vi "SHG_scattering_control.vi"() -> ()   [LabVIEW 2017]
uses:
  <instrlib>/Keithley 2200 Series/Keithley 2200 Series.lvlib
panel:
  in  "batch_bck location":path
  in  "batch_shg location":path
  in  "Take_bck_scan.exe location":path
  in  "Exposure Time (s)":dbl format="%#_13g"
  in  "Ouput Polarization (P_out OR S_out)":string
  in  "SHG_scat_scan.exe location":path
  in  "Power Supply":refnum<visa-resource-name>
  in  "Angle Resolution\n(Degrees per step)":i32
  in  "Min Angle":i32
  in  "Max Angle":i32
  in  "Number of Accum.":i32
  in  "S_in":bool=TRUE
  in  "P_in":bool=TRUE
  in  "System":string
  # "These file paths will be set to default positions"
  # "Data File parameters\n(Files save as: \nSystem_outputPol_inputPol_##_degrees_date)"
  # "Scan Inputs"
  # "The acceptable range is from\n-90 to 110 degrees"
  # "Polarizations to use (all nonrepetitive\n combinations will be scanned)"
  # "NOTE: If you make an emergency stop you must reset the stages manually from the terminal or controller unit!"
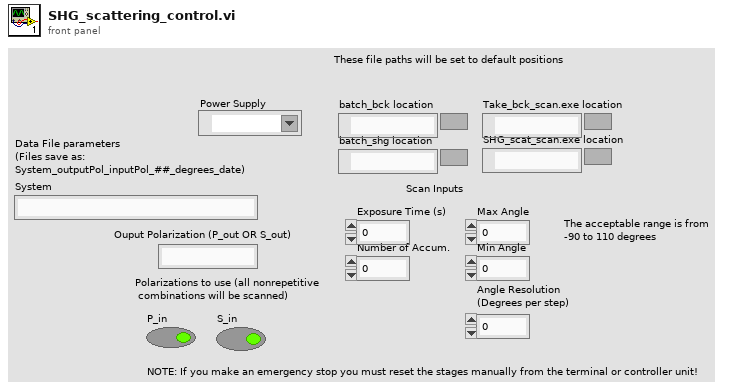
[diagram p1: front panel]
types:
  T1 = cluster{"connection TCP":refnum<k5>, "LogTo File":bool, "Log File refnum":refnum<file>, "no error if error log":bool}
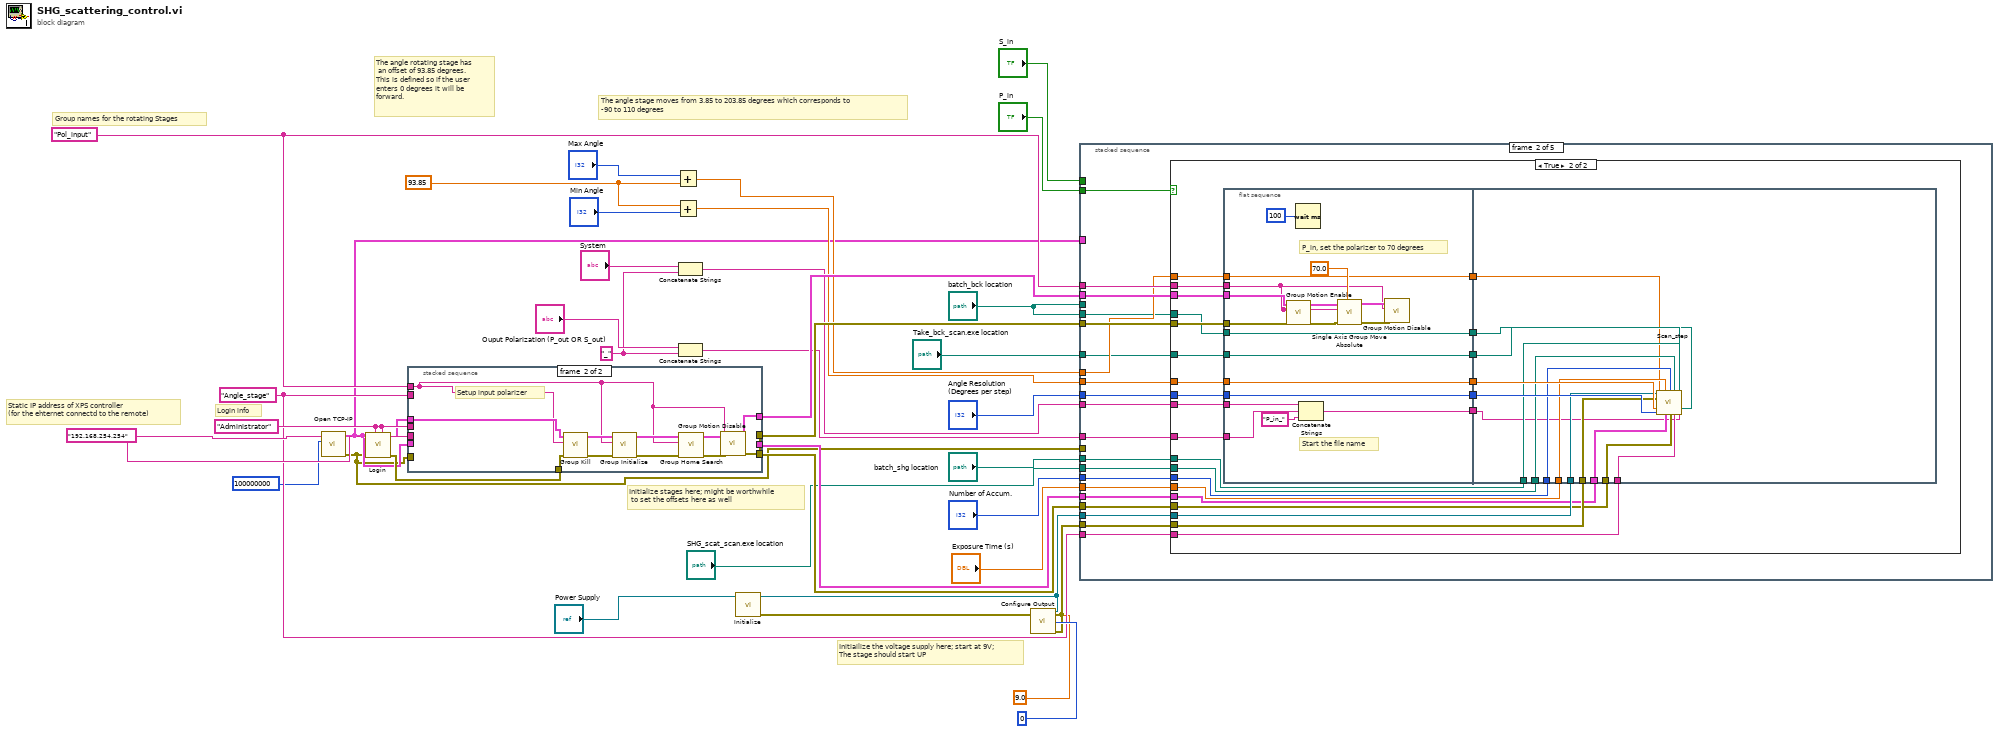
[diagram p0: block diagram]
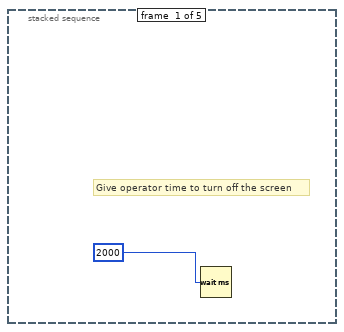
[diagram p2: hidden frame]
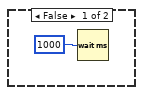
[diagram p3: hidden frame]
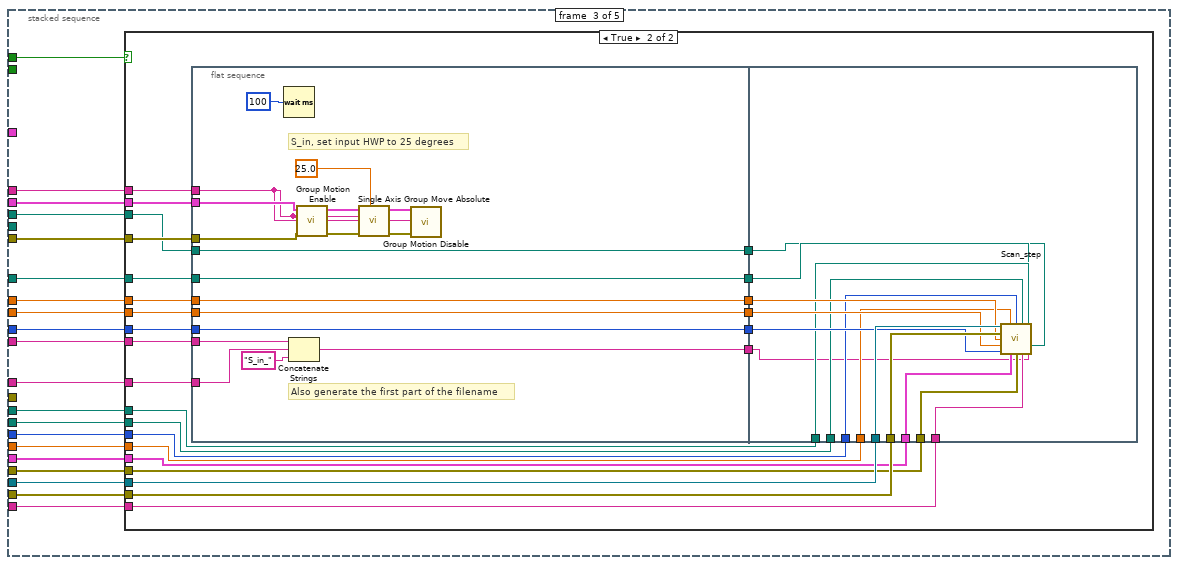
[diagram p4: hidden frame]
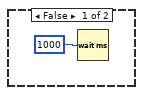
[diagram p5: hidden frame]
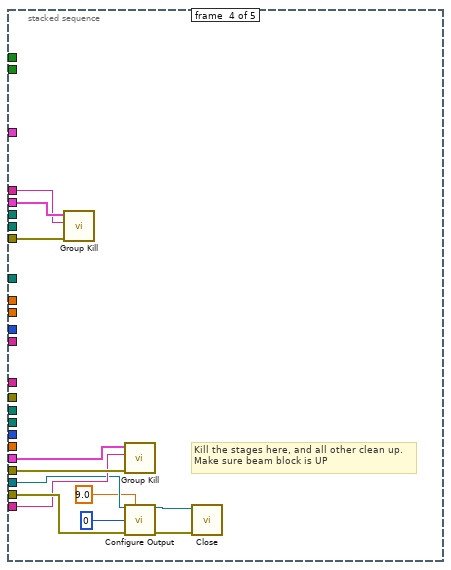
[diagram p6: hidden frame]
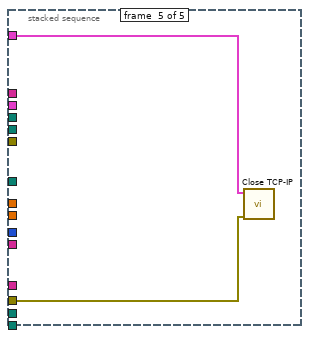
[diagram p7: hidden frame]
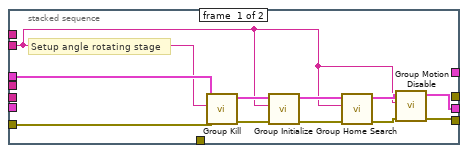
[diagram p8: hidden frame]
diagram:
  w9 = "_"
  w21 = 93.85
  w37 = "Administrator"
  w29 = "Angle_stage"
  w26 = "Pol_input"
  w36 = "192.168.254.254"
  # "The angle stage moves from 3.85 to 203.85 degrees which corresponds to \n-90 to 110 degrees"
  # "The angle rotating stage has\n an offset of 93.85 degrees.\nThis is defined so if the user \nenters 0 degrees it will be \nforward."
  # "Login info"
  # "Initiailize the voltage supply here; start at 9V;\nThe stage should start UP"
  # "Initialize stages here; might be worthwhile\n to set the offsets here as well"
  # "Group names for the rotating Stages"
  # "Static IP address of XPS controller\n(for the ehternet connectd to the remote)"
  n1 = call <userlib>:"Open TCP-IP.vi"("timeout ms (60000)"=100000000, "IP address"=w36) -> ("error out"=w1:errorcluster, "Connection ID"=w2:T1)  [unwired: 7 in, 1 out]
  n2 = call <userlib>:"Login.vi"("Password"=w37, "User"=w37, "error in (no error)"=w1, "connection ID in"=w2) -> ("error out"=w6:errorcluster, "connection ID out"=w5:T1)  [unwired: 5 in, 1 out]
  n3 = stacked-sequence {
    tunnel: w29 -> [w38 _]
    tunnel: w26 -> [_ w49]
    tunnel: w37 -> [_ _]
    tunnel: w36 -> [_ _]
    tunnel: [_ w51] -> w31
    tunnel: [_ w50] -> w30
    tunnel: [w40 _] -> w28
    tunnel: [w39 _] -> w27
    tunnel: w1 -> [w43 _]
    tunnel: w2 -> [_ _]
    tunnel: w6 -> [_ w55]
    tunnel: w5 -> [w44 w54]
    frame #0 {
      # "Setup angle rotating stage"
      n4 = call <userlib>:"Group Kill.vi"("error in (no error)"=w43, "Group Name (250 c max)"=w38, "connection ID in"=w44) -> ("error out"=w47:errorcluster, "connection ID out"=w45:T1)  [unwired: 6 in, 1 out]
      n5 = call <userlib>:"Group Initialize.vi"("error in (no error)"=w47, "Group Name (250 c max)"=w38, "connection ID in"=w45) -> ("error out"=w48:errorcluster, "connection ID out"=w46:T1)  [unwired: 6 in, 1 out]
      n6 = call <userlib>:"Group Home Search.vi"("error in (no error)"=w48, "Group Name (250 c max)"=w38, "connection ID in"=w46) -> ("error out"=w41:errorcluster, "connection ID out"=w42:T1)  [unwired: 6 in, 1 out]
      n7 = call <userlib>:"Group Motion Disable.vi"("error in (no error)"=w41, "Group Name (250 c max)"=w38, "connection ID in"=w42) -> ("error out"=w39:errorcluster, "connection ID out"=w40:T1)  [unwired: 6 in, 1 out]
    }
    frame #1 {
      # "Setup input polarizer"
      n8 = call <userlib>:"Group Kill.vi"("error in (no error)"=w55, "Group Name (250 c max)"=w49, "connection ID in"=w54) -> ("error out"=w57:errorcluster, "connection ID out"=w59:T1)  [unwired: 6 in, 1 out]
      n9 = call <userlib>:"Group Initialize.vi"("error in (no error)"=w57, "Group Name (250 c max)"=w49, "connection ID in"=w59) -> ("error out"=w56:errorcluster, "connection ID out"=w58:T1)  [unwired: 6 in, 1 out]
      n10 = call <userlib>:"Group Home Search.vi"("error in (no error)"=w56, "Group Name (250 c max)"=w49, "connection ID in"=w58) -> ("error out"=w52:errorcluster, "connection ID out"=w53:T1)  [unwired: 6 in, 1 out]
      n11 = call <userlib>:"Group Motion Disable.vi"("error in (no error)"=w52, "Group Name (250 c max)"=w49, "connection ID in"=w53) -> ("error out"=w50:errorcluster, "connection ID out"=w51:T1)  [unwired: 6 in, 1 out]
    }
  }
  n12 = Add(x="Max Angle", y=w21) -> (x+y=w3:dbl)
  n13 = Add(x=w21, y="Min Angle") -> (x+y=w20:dbl)
  n14 = Concatenate Strings("System", w9) -> (w11:string)
  n15 = Concatenate Strings("Ouput Polarization (P_out OR S_out)", w9) -> (w8:string)
  n16 = call <instrlib>:"Initialize.vi"("VISA resource name"="Power Supply") -> ("error out"=w24:errorcluster, "VISA resource name out"=w25:refnum<visa-resource-name>)  [unwired: 9 in]
  n17 = call <instrlib>:"Configure Output.vi"("VISA resource name"=w25, "Manual Range(0.00)"=9.0, "Function(0:Voltage)"=0, "error in (no error)"=w24) -> ()  [unwired: 10 in, 2 out]
  n18 = stacked-sequence {
    tunnel: "P_in" -> [_ w80 _ _ _]
    tunnel: "S_in" -> [_ _ w159 _ _]
    tunnel: w31 -> [_ w79 w153 w228 _]
    tunnel: w30 -> [_ w78 w152 w227 _]
    tunnel: w26 -> [_ w77 w151 w226 _]
    tunnel: w29 -> [_ w69 w148 w223 _]
    tunnel: w28 -> [_ w71 w150 w225 _]
    tunnel: w27 -> [_ w70 w149 w224 _]
    tunnel: w25 -> [_ w76 w158 w222 _]
    tunnel: w24 -> [_ w75 w157 w229 _]
    tunnel: w3 -> [_ w74 w154 _ _]
    tunnel: w20 -> [_ w73 w155 _ _]
    tunnel: "Angle Resolution\n(Degrees per step)" -> [_ w72 w156 _ _]
    tunnel: "Exposure Time (s)" -> [_ w68 w147 _ _]
    tunnel: "Number of Accum." -> [_ w67 w146 _ _]
    tunnel: "SHG_scat_scan.exe location" -> [_ w66 w144 _ _]
    tunnel: "batch_shg location" -> [_ w65 w145 _ _]
    tunnel: "Take_bck_scan.exe location" -> [_ w64 w143 _ _]
    tunnel: "batch_bck location" -> [_ w63 _ _ _]
    tunnel: "batch_bck location" -> [_ _ w142 _ _]
    tunnel: w11 -> [_ w62 w141 _ _]
    tunnel: w8 -> [_ w61 w140 _ _]
    tunnel: w2 -> [_ _ _ _ w232]
    tunnel: w1 -> [_ _ _ _ w231]
    frame #0 {
      # "Give operator time to turn off the screen"
      n19 = Wait (ms)(milliseconds to wait=2000) -> ()  [unwired: 1 out]
    }
    frame #1 {
      n20 = case shown="True" w80 {
        tunnel: w79 -> [_ w106]
        tunnel: w78 -> [_ w105]
        tunnel: w77 -> [_ w104]
        tunnel: w76 -> [_ w98]
        tunnel: w75 -> [_ w99]
        tunnel: w74 -> [_ w82]
        tunnel: w73 -> [_ w100]
        tunnel: w72 -> [_ w102]
        tunnel: w71 -> [_ w97]
        tunnel: w70 -> [_ w96]
        tunnel: w69 -> [_ w95]
        tunnel: w68 -> [_ w94]
        tunnel: w67 -> [_ w93]
        tunnel: w66 -> [_ w92]
        tunnel: w65 -> [_ w91]
        tunnel: w64 -> [_ w90]
        tunnel: w63 -> [_ w88]
        tunnel: w62 -> [_ w86]
        tunnel: w61 -> [_ w85]
        frame False {
          n21 = Wait (ms)(milliseconds to wait=1000) -> ()  [unwired: 1 out]
        }
        frame True {
          n22 = flat-sequence {
            tunnel: w106 -> [w111]
            tunnel: w105 -> [w110]
            tunnel: w104 -> [w107]
            tunnel: [w122] -> w103
            tunnel: w102 -> [w122]
            tunnel: [w121] -> w101
            tunnel: w100 -> [w121]
            tunnel: w90 -> [w120]
            tunnel: [w120] -> w89
            tunnel: w88 -> [w119]
            tunnel: [w119] -> w87
            tunnel: w86 -> [w118]
            tunnel: w85 -> [w117]
            tunnel: [w115] -> w84
            tunnel: [w114] -> w83
            tunnel: w82 -> [w114]
            tunnel: w103 -> [w139]
            tunnel: w101 -> [w138]
            tunnel: w99 -> [w137]
            tunnel: w98 -> [w136]
            tunnel: w97 -> [w135]
            tunnel: w96 -> [w134]
            tunnel: w95 -> [w133]
            tunnel: w94 -> [w132]
            tunnel: w93 -> [w131]
            tunnel: w92 -> [w130]
            tunnel: w91 -> [w129]
            tunnel: w89 -> [w128]
            tunnel: w87 -> [w127]
            tunnel: w84 -> [w126]
            tunnel: w83 -> [w125]
            frame #0 {
              # "Start the file name"
              # "P_in, set the polarizer to 70 degrees"
              n23 = call <userlib>:"Group Motion Enable.vi"("error in (no error)"=w110, "Group Name (250 c max)"=w107, "connection ID in"=w111) -> ("error out"=w109:errorcluster, "connection ID out"=w113:T1)  [unwired: 6 in, 1 out]
              n24 = Wait (ms)(milliseconds to wait=100) -> ()  [unwired: 1 out]
              n25 = Concatenate Strings(w118, w117, "P_in_") -> (w115:string)
              n26 = call <userlib>:"Single Axis Group Move Absolute.vi"("Target Position (units)"=70.0, "error in (no error)"=w109, "SingleAxis Group  Name (250 c max)"=w107, "connection ID in"=w113) -> ("error out"=w108:errorcluster, "connection ID out"=w112:T1)  [unwired: 5 in, 1 out]
              n27 = call <userlib>:"Group Motion Disable.vi"("error in (no error)"=w108, "Group Name (250 c max)"=w107, "connection ID in"=w112) -> ()  [unwired: 6 in, 3 out]
            }
            frame #1 {
              n28 = call "Scan_step.vi"("Power Supply"=w136, "Exposure Time (s)"=w132, "Number of Accumulations"=w131, "Location of SHG_scat_scan.exe"=w130, "Location of batch_shg"=w129, "Error in (Power Supply)"=w137, "Location of Take_bck_scan.exe"=w128, "Max Angle"=w125, "Min Angle"=w138, "Location of batch_bck"=w127, "Angle Resolution"=w139, "Stage Connection in"=w135, "Error in (Stage)"=w134, "Group Name"=w133, "DataFile name"=w126) -> ()  [unwired: 1 in]
            }
          }
        }
      }
    }
    frame #2 {
      n29 = case shown="True" w159 {
        tunnel: w158 -> [_ w185]
        tunnel: w157 -> [_ w184]
        tunnel: w156 -> [_ w182]
        tunnel: w155 -> [_ w180]
        tunnel: w154 -> [_ w178]
        tunnel: w153 -> [_ w177]
        tunnel: w152 -> [_ w176]
        tunnel: w151 -> [_ w175]
        tunnel: w150 -> [_ w174]
        tunnel: w149 -> [_ w173]
        tunnel: w148 -> [_ w172]
        tunnel: w147 -> [_ w171]
        tunnel: w146 -> [_ w170]
        tunnel: w145 -> [_ w169]
        tunnel: w144 -> [_ w168]
        tunnel: w143 -> [_ w167]
        tunnel: w142 -> [_ w165]
        tunnel: w141 -> [_ w163]
        tunnel: w140 -> [_ w162]
        frame False {
          n30 = Wait (ms)(milliseconds to wait=1000) -> ()  [unwired: 1 out]
        }
        frame True {
          n31 = flat-sequence {
            tunnel: [w201] -> w183
            tunnel: w182 -> [w201]
            tunnel: [w200] -> w181
            tunnel: w180 -> [w200]
            tunnel: [w199] -> w179
            tunnel: w178 -> [w199]
            tunnel: w177 -> [w188]
            tunnel: w176 -> [w187]
            tunnel: w175 -> [w186]
            tunnel: w167 -> [w198]
            tunnel: [w198] -> w166
            tunnel: w165 -> [w197]
            tunnel: [w197] -> w164
            tunnel: w163 -> [w196]
            tunnel: w162 -> [w195]
            tunnel: [w193] -> w161
            tunnel: w185 -> [w218]
            tunnel: w184 -> [w217]
            tunnel: w183 -> [w216]
            tunnel: w181 -> [w215]
            tunnel: w179 -> [w214]
            tunnel: w174 -> [w213]
            tunnel: w173 -> [w212]
            tunnel: w172 -> [w211]
            tunnel: w171 -> [w210]
            tunnel: w170 -> [w209]
            tunnel: w169 -> [w208]
            tunnel: w168 -> [w207]
            tunnel: w166 -> [w206]
            tunnel: w164 -> [w205]
            tunnel: w161 -> [w204]
            frame #0 {
              # "Also generate the first part of the filename"
              # "S_in, set input HWP to 25 degrees"
              n32 = Wait (ms)(milliseconds to wait=100) -> ()  [unwired: 1 out]
              n33 = Concatenate Strings(w196, w195, "S_in_") -> (w193:string)
              n34 = call <userlib>:"Group Motion Enable.vi"("error in (no error)"=w187, "Group Name (250 c max)"=w186, "connection ID in"=w188) -> ("error out"=w190:errorcluster, "connection ID out"=w191:T1)  [unwired: 6 in, 1 out]
              n35 = call <userlib>:"Single Axis Group Move Absolute.vi"("Target Position (units)"=25.0, "error in (no error)"=w190, "SingleAxis Group  Name (250 c max)"=w186, "connection ID in"=w191) -> ("error out"=w189:errorcluster, "connection ID out"=w192:T1)  [unwired: 5 in, 1 out]
              n36 = call <userlib>:"Group Motion Disable.vi"("error in (no error)"=w189, "Group Name (250 c max)"=w186, "connection ID in"=w192) -> ()  [unwired: 6 in, 3 out]
            }
            frame #1 {
              n37 = call "Scan_step.vi"("Power Supply"=w218, "Exposure Time (s)"=w210, "Number of Accumulations"=w209, "Location of SHG_scat_scan.exe"=w207, "Location of batch_shg"=w208, "Error in (Power Supply)"=w217, "Location of Take_bck_scan.exe"=w206, "Max Angle"=w214, "Min Angle"=w215, "Location of batch_bck"=w205, "Angle Resolution"=w216, "Stage Connection in"=w213, "Error in (Stage)"=w212, "Group Name"=w211, "DataFile name"=w204) -> ()  [unwired: 1 in]
            }
          }
        }
      }
    }
    frame #3 {
      # "Kill the stages here, and all other clean up.\nMake sure beam block is UP"
      n38 = call <userlib>:"Group Kill.vi"("error in (no error)"=w227, "Group Name (250 c max)"=w226, "connection ID in"=w228) -> ()  [unwired: 6 in, 3 out]
      n39 = call <userlib>:"Group Kill.vi"("error in (no error)"=w224, "Group Name (250 c max)"=w223, "connection ID in"=w225) -> ()  [unwired: 6 in, 3 out]
      n40 = call <instrlib>:"Configure Output.vi"("VISA resource name"=w222, "Manual Range(0.00)"=9.0, "Function(0:Voltage)"=0, "error in (no error)"=w229) -> ("VISA resource name out"=w221:refnum<visa-resource-name>, "error out"=w220:errorcluster)  [unwired: 10 in]
      n41 = call <instrlib>:"Close.vi"("error in (no error)"=w220, "VISA resource name"=w221) -> ()  [unwired: 9 in, 1 out]
    }
    frame #4 {
      n42 = call <userlib>:"Close TCP-IP.vi"("error in (no error)"=w231, "connection ID in"=w232) -> ()  [unwired: 9 in, 1 out]
    }
  }
